vi "Read Voltage.vi"(8 "error in (no error)":errorcluster, 11 "Voltmeter CFG in":refnum<class "Voltmeter CFG.lvclass">) -> (0 "error out":errorcluster, 2 "Voltage":dbl format="%#_g V", 3 "Voltmeter CFG out":refnum<class "Voltmeter CFG.lvclass">)   [LabVIEW 2023, in "PXIe-5172.lvlib" / "Voltmeter CFG.lvclass"]
uses:
  Voltmeter CFG.lvclass
  <vilib>/Analysis/baseanly.llb/Mean (DBL).vi
  Voltmeter CFG.lvclass/Voltmeter CFG.ctl
  <vilib>/Analysis/NI_AALBase.lvlib
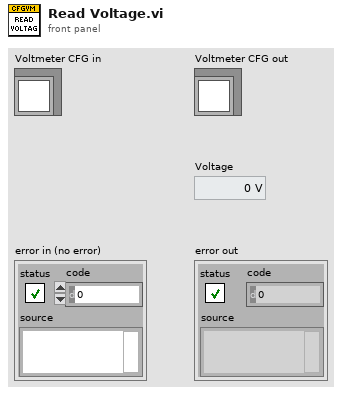
[diagram p1: front panel]
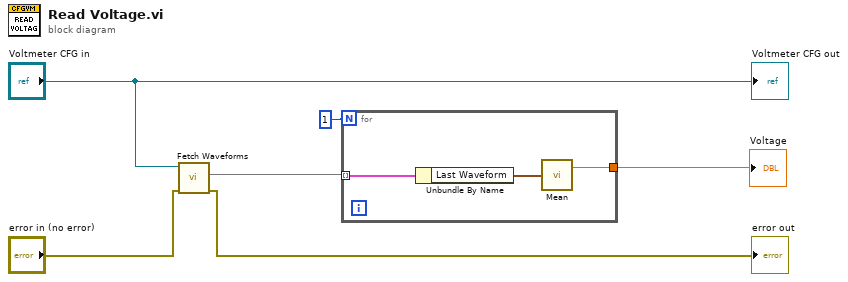
[diagram p0: block diagram]
diagram:
  n1 = call-dynamic "Fetch Waveforms.vi"("error in"="error in (no error)", "object in"="Voltmeter CFG in") -> ("error out"=→"error out":errorcluster, "Last Waveforms"=w4:map{u8, waveform(dbl)})  [unwired: 7 in, 1 out]
  n2 = for {
    N: 1 -> [_]
    tunnel: [w9] -> w5
    tunnel: w4 -> [w8] mode=indexing
    n3 = Unbundle By Name(w8) -> ("Last Waveform"=w7:waveform(dbl))
    n4 = call-poly <vilib>:"Mean.vi"("X"=w7) -> ("mean"=w9:dbl)  [unwired: 1 out]
  }
  "Voltage" <- w5
  "Voltmeter CFG out" <- "Voltmeter CFG in"
